vi "Client 1 - Copy1.vi"() -> ()   [LabVIEW 2017]
uses:
  <vilib>/Analysis/Matrix/Datatypes/RealMatrix.ctl
  <vilib>/Analysis/Matrix/NI_Matrix.lvlib
panel:
  out "decimal integer string":string[][](array[string])
  in  "Matrix 1":T1
  out "bytes written":i32
  out "data string":string
  in  "stop":bool
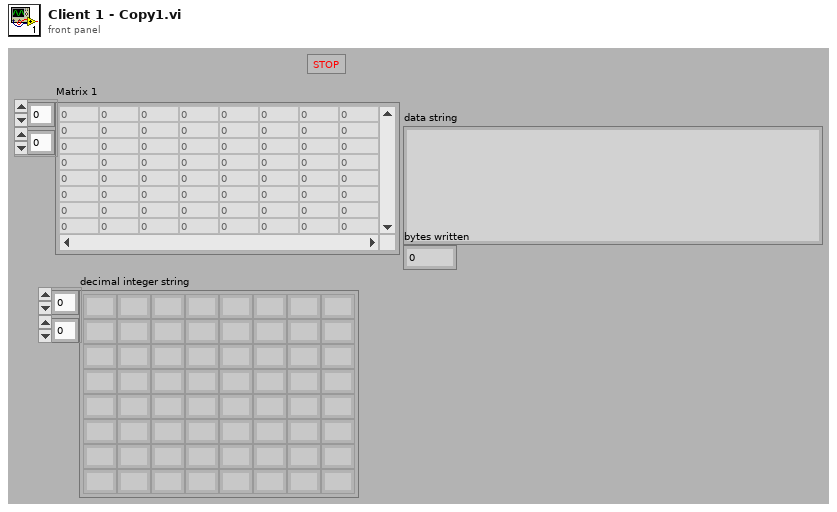
[diagram p1: front panel]
types:
  T1 = typedef "NI_Matrix.lvlib/RealMatrix.ctl" = dbl[][]
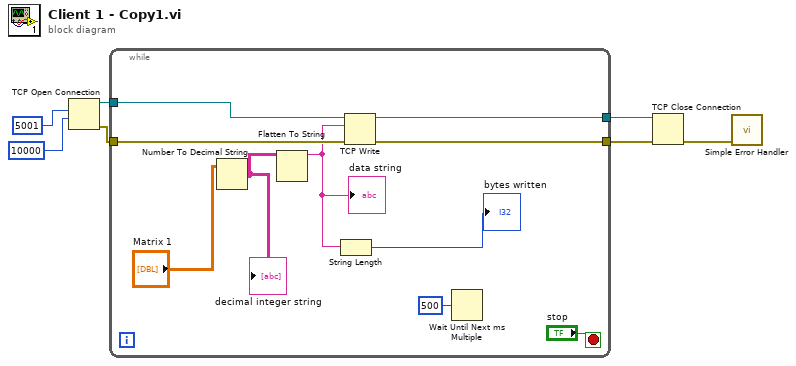
[diagram p0: block diagram]
diagram:
  n1 = TCP Open Connection(remote port or service name=u16 5001, timeout ms (60000)=10000) -> (connection ID=w5:refnum<k5>, error out=w4:errorcluster)  [unwired: 3 in]
  n2 = while {
    tunnel: w5 -> [w16]
    tunnel: w4 -> [w15]
    tunnel: [w14] -> w2
    tunnel: [w13] -> w1
    stop <- "stop" stop-if-true
    n3 = Number To Decimal String(number="Matrix 1") -> (decimal integer string=w10:string[][])  [unwired: 1 in]
    "decimal integer string" <- w10
    n4 = Flatten To String(anything=w10) -> (data string=w9:string)  [unwired: 3 in, 2 out]
    "data string" <- w9
    n5 = String Length(string=w9) -> (length=→"bytes written":i32)
    n6 = TCP Write(connection ID=w16, data in=w9, error in (no error)=w15) -> (connection ID out=w14:refnum<k5>, error out=w13:errorcluster)  [unwired: 1 in, 1 out]
    n7 = Wait Until Next ms Multiple(millisecond multiple=u32 500) -> ()  [unwired: 1 out]
  }
  n8 = TCP Close Connection(connection ID=w2, error in (no error)=w1) -> (error out=w3:errorcluster)  [unwired: 1 in, 1 out]
  n9 = call <vilib>:"Simple Error Handler.vi"("error in (no error)"=w3) -> ()  [unwired: 4 in, 5 out]
